vi "Focus PUSH.vi"(9 "action":string="STATUS", 11 "clientTransactionId":i64) -> (2 "pushedMessage":string)   [LabVIEW 2018]
uses:
  Global_Telescopio.vi
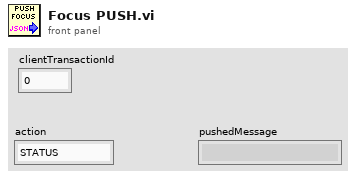
[diagram p1: front panel]
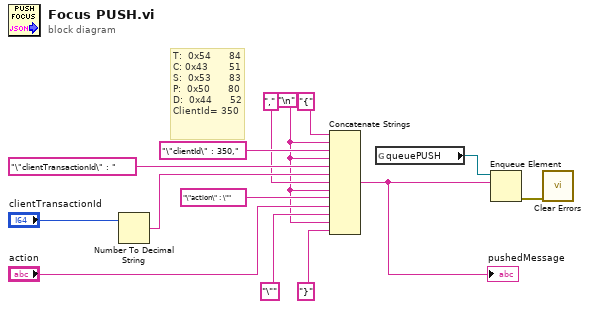
[diagram p0: block diagram]
diagram:
  w5 = "\n"
  # "T:  0x54      84\nC: 0x43       51\nS:  0x53      83\nP:  0x50      80\nD:  0x44      52\nClientId= 350"
  n1 = Number To Decimal String(number="clientTransactionId") -> (decimal integer string=w10:string)  [unwired: 1 in]
  n2 = Concatenate Strings("{" ("controller"), w5, "\"clientId\" : 350," ("controller"), w5, "\"clientTransactionId\" : " ("controller"), w10, "," ("controller"), w5, "\"action\" : \"" ("controller"), "action", "\"" ("controller"), w5, "}" ("controller")) -> (w3:string)
  "pushedMessage" <- w3
  n3 = global read "Global_Telescopio.vi" "queuePUSH"() -> (w2:refnum<queue>)
  n4 = Enqueue Element(queue=w2, element=w3) -> (error out=w1:errorcluster)  [unwired: 2 in, 2 out]
  n5 = call <vilib>:"Clear Errors.vi"("error in (no error)"=w1) -> ()  [unwired: 5 in, 2 out]
